vi "Auto_Gain.vi"(8 "error in (no error)":errorcluster, 10 "Auto gain":bool, 11 ".NET Refnum in":refnum<k24>) -> (0 "error out":errorcluster, 3 ".NET Refnum out":refnum<k24>)   [LabVIEW 2021]
uses:
  C:/Program Files/Thorlabs/Scientific Imaging/ThorCam/uc480DotNet.dll
  Program Files/Thorlabs/Scientific Imaging/ThorCam/uc480DotNet.dll
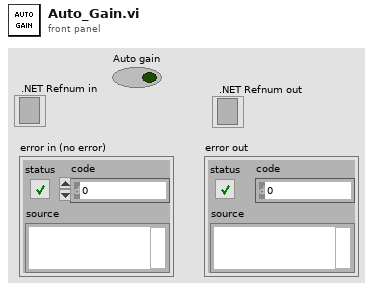
[diagram p1: front panel]
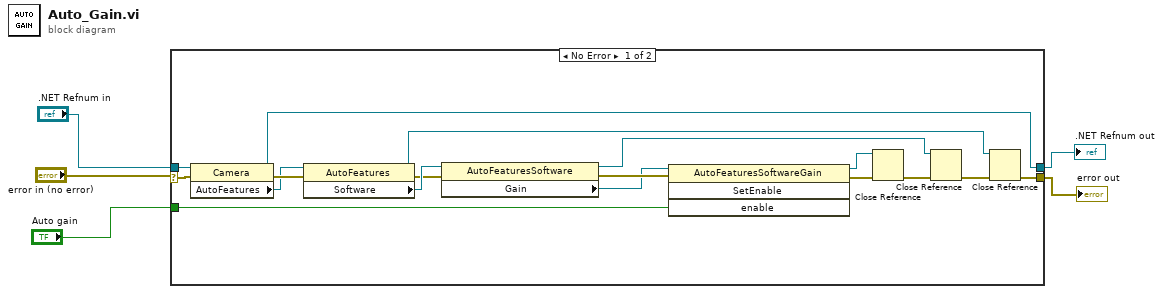
[diagram p0: block diagram]
diagram:
  n1 = case shown="No Error" "error in (no error)" {
    selector: "error in (no error)" -> [w7 w23]
    tunnel: [w22 w23] -> w5
    tunnel: ".NET Refnum in" -> [w9 w24]
    tunnel: "Auto gain" -> [w8 _]
    tunnel: [w6 w24] -> w1
    frame No Error {
      n2 = property class="Camera"(reference=w9, error in=w7) -> (reference out=w6:refnum<k24>, error out=w11:errorcluster, "AutoFeatures"=w10:refnum<k24>)
      n3 = property class="AutoFeatures"(reference=w10, error in=w11) -> (reference out=w17:refnum<k24>, error out=w12:errorcluster, "Software"=w13:refnum<k24>)
      n4 = property class="AutoFeaturesSoftware"(reference=w13, error in=w12) -> (reference out=w15:refnum<k24>, error out=w21:errorcluster, "Gain"=w18:refnum<k24>)
      n5 = invoke class="AutoFeaturesSoftwareGain" method="SetEnable"(reference=w18, error in=w21, "enable"=w8) -> (reference out=w20:refnum<k24>, error out=w19:errorcluster)  [unwired: 1 in, 2 out]
      n6 = Close Reference(reference=w20, error in (no error)=w19) -> (error out=w14:errorcluster)
      n7 = Close Reference(reference=w15, error in (no error)=w14) -> (error out=w16:errorcluster)
      n8 = Close Reference(reference=w17, error in (no error)=w16) -> (error out=w22:errorcluster)
    }
    frame Error {
    }
  }
  "error out" <- w5
  ".NET Refnum out" <- w1
